vi "Variant to Array of Variants.vi"(8 "error in (no error)":errorcluster, 11 "value":variant) -> (0 "error out":errorcluster, 3 "Variant (1D array)":variant[](array[variant]))   [LabVIEW 2019, in "Control Experiment.lvclass"]
uses:
  Control Experiment.lvclass
  <vilib>/Utility/Data Type/NI_Data Type.lvlib
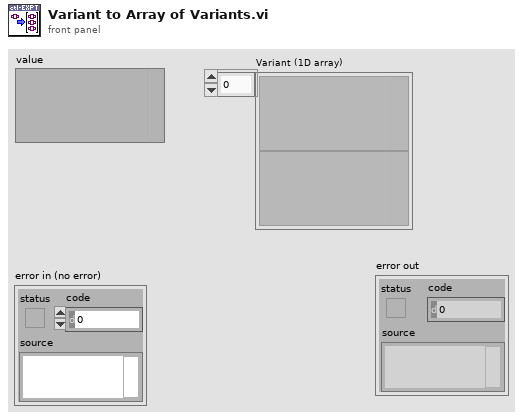
[diagram p1: front panel]
types:
  T1 = typedef "NI_Data Type.lvlib/Data Type.ctl" = enum8{"Invalid Type", "Void", "I8", "I16", "I32", "I64", "U8", "U16", "U32", "U64", "Single Float", "Double Float", "Extended Float", "Single Complex", "Double Complex", "Extended Complex", "Enum U8", "Enum U16", "Enum U32", "Enum U64", "Single Float With Unit", "Double Float With Unit", "Extended Float With Unit", "Single Complex with Unit", "Double Complex with Unit", "Extended Complex with Unit", "Boolean", "String", "Path", "Picture", "Tag", "Array", "Cluster", "Variant", "LV Variant", "Waveform", "Timestamp", "Digital Waveform", "Digital Data", "ExpressData", "Refnum", "External Data", "VI", "Poly VI", "LabVIEW Class Instance", "Fixed Point", "Set Collection", "Map Collection"}
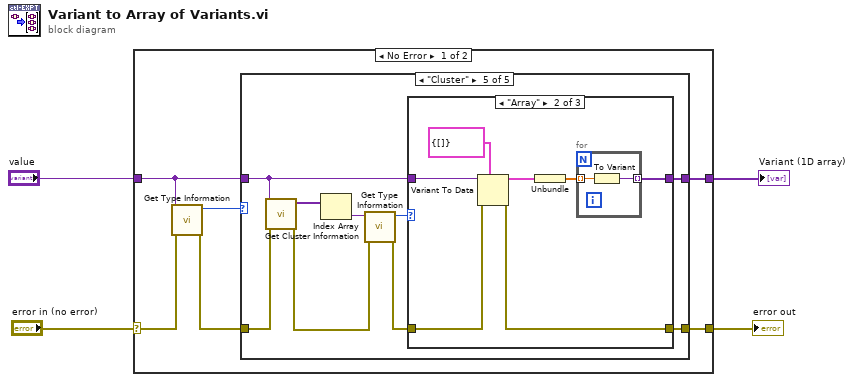
[diagram p0: block diagram]
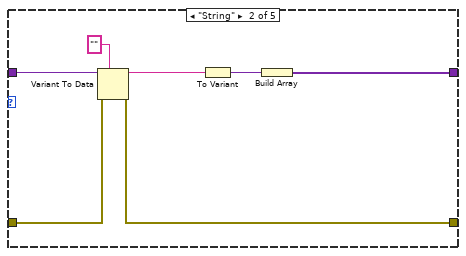
[diagram p3: hidden frame]
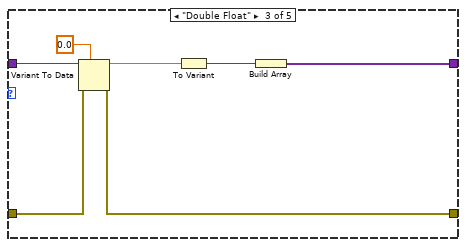
[diagram p4: hidden frame]
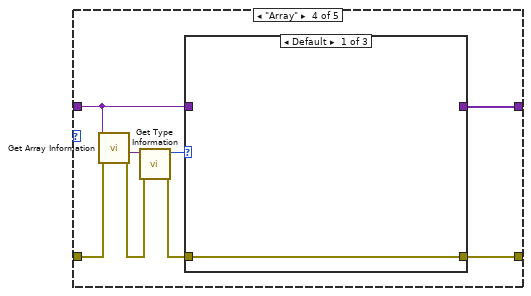
[diagram p5: hidden frame]
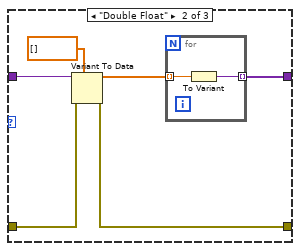
[diagram p6: hidden frame]
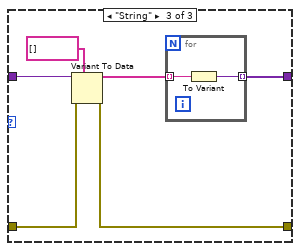
[diagram p7: hidden frame]
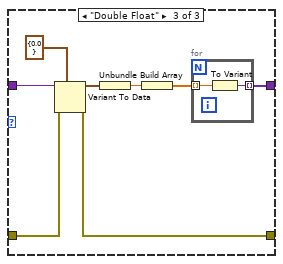
[diagram p9: hidden frame]
diagram:
  n1 = case shown="No Error" "error in (no error)" {
    selector: "error in (no error)" -> [w7 w80]
    tunnel: [w8 w80] -> w3
    tunnel: "value" -> [w5 _]
    tunnel: [w9 _] -> w1
    frame No Error {
      n2 = call <vilib>:"Get Type Information.vi"("error in (no error)"=w7, "variant"=w5) -> ("error out"=w6:errorcluster, "type"=w10:T1)  [unwired: 5 in, 3 out]
      n3 = case shown="\"Cluster\"" w10 {
        tunnel: [_ w12 w19 w32 w54] -> w9
        tunnel: w5 -> [_ w17 w25 w31 w52]
        tunnel: w6 -> [w11 w15 w24 w30 w59]
        tunnel: [w11 w16 w22 w33 w53] -> w8
        frame Default {
        }
        frame "String" {
          n4 = Variant To Data(error in=w15, type="", Variant=w17) -> (data=w14:string, error out=w16:errorcluster)
          n5 = To Variant(anything=w14) -> (Variant=w13:variant)
          n6 = Build Array(w13) -> (w12:variant[])
        }
        frame "Double Float" {
          n7 = Variant To Data(error in=w24, type=0.0, Variant=w25) -> (data=w21:dbl, error out=w22:errorcluster)
          n8 = To Variant(anything=w21) -> (Variant=w20:variant)
          n9 = Build Array(w20) -> (w19:variant[])
        }
        frame "Array" {
          n10 = call <vilib>:"Get Array Information.vi"("error in (no error)"=w30, "variant"=w31) -> ("error out"=w27:errorcluster, "array element data type"=w29:variant)  [unwired: 6 in, 2 out]
          n11 = call <vilib>:"Get Type Information.vi"("error in (no error)"=w27, "variant"=w29) -> ("error out"=w26:errorcluster, "type"=w28:T1)  [unwired: 5 in, 3 out]
          n12 = case shown="Default" w28 {
            tunnel: [w34 w39 w47] -> w33
            tunnel: [_ w37 w45] -> w32
            tunnel: w31 -> [_ w36 w44]
            tunnel: w26 -> [w34 w35 w43]
            frame Default {
            }
            frame "Double Float" {
              n13 = Variant To Data(error in=w35, type=dbl[] [], Variant=w36) -> (data=w38:dbl[], error out=w39:errorcluster)
              n14 = for {
                tunnel: w38 -> [w42] mode=indexing
                tunnel: [w41] -> w37 mode=indexing
                n15 = To Variant(anything=w42) -> (Variant=w41:variant)
              }
            }
            frame "String" {
              n16 = Variant To Data(error in=w43, type=string[] [], Variant=w44) -> (data=w46:string[], error out=w47:errorcluster)
              n17 = for {
                tunnel: w46 -> [w50] mode=indexing
                tunnel: [w49] -> w45 mode=indexing
                n18 = To Variant(anything=w50) -> (Variant=w49:variant)
              }
            }
          }
        }
        frame "Cluster" {
          n19 = call <vilib>:"Get Cluster Information.vi"("error in (no error)"=w59, "variant"=w52) -> ("error out"=w57:errorcluster, "cluster elements"=w58:variant[])  [unwired: 8 in]
          n20 = Index Array(array=w58) -> (element=w56:variant)  [unwired: 1 in]
          n21 = call <vilib>:"Get Type Information.vi"("error in (no error)"=w57, "variant"=w56) -> ("error out"=w51:errorcluster, "type"=w55:T1)  [unwired: 5 in, 3 out]
          n22 = case shown="\"Array\"" w55 {
            tunnel: [_ w62 w70] -> w54
            tunnel: w52 -> [_ w66 w76]
            tunnel: w51 -> [w60 w65 w75]
            tunnel: [w60 w61 w73] -> w53
            frame Default {
            }
            frame "Array" {
              n23 = Variant To Data(error in=w65, type=cluster{dbl[]} {[]}, Variant=w66) -> (data=w67:cluster{dbl[]}, error out=w61:errorcluster)
              n24 = Unbundle(w67) -> (w63:dbl[])
              n25 = for {
                tunnel: w63 -> [w69] mode=indexing
                tunnel: [w68] -> w62 mode=indexing
                n26 = To Variant(anything=w69) -> (Variant=w68:variant)
              }
            }
            frame "Double Float" {
              n27 = Variant To Data(error in=w75, type=cluster{dbl} {0.0}, Variant=w76) -> (data=w77:cluster{dbl}, error out=w73:errorcluster)
              n28 = Unbundle(w77) -> (w71:dbl)
              n29 = Build Array(w71) -> (w74:dbl[])
              n30 = for {
                tunnel: w74 -> [w79] mode=indexing
                tunnel: [w78] -> w70 mode=indexing
                n31 = To Variant(anything=w79) -> (Variant=w78:variant)
              }
            }
          }
        }
      }
    }
    frame Error {
    }
  }
  "error out" <- w3
  "Variant (1D array)" <- w1
